vi "CSTK_Icon_Creator_Insert_UpdateImageData.vi"(6 "图片数据输入":T1, 8 "error in (no error)":errorcluster, 11 "图片输入":picture) -> (0 "error out":errorcluster, 3 "图片输出":picture, 4 "图片数据输出":T1)   [LabVIEW 2015, in "CSTK_Icon Creator.lvlib"]
uses:
  CSTK_Icon Creator.lvlib
  <vilib>/picture/picture.llb/imagedata.ctl
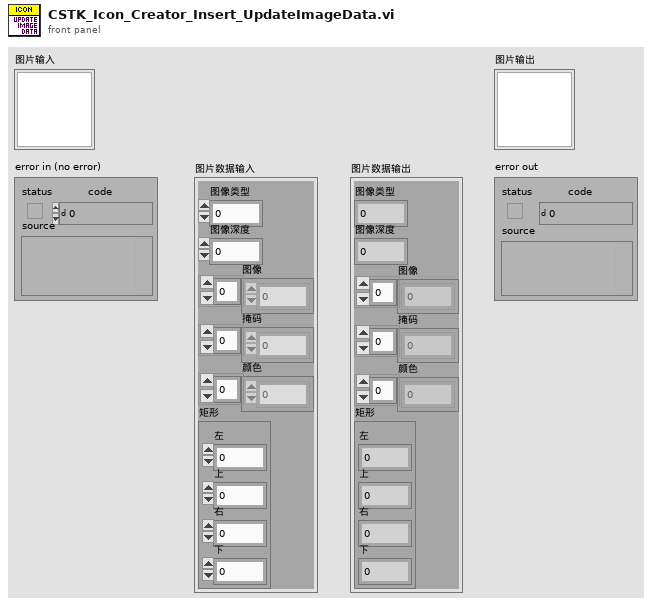
[diagram p1: front panel]
types:
  T1 = typedef "imagedata.ctl" = cluster{"image type":i32, "image depth":i32, "image":u8[], "mask":u8[], "colors":u32[], "Rectangle":cluster{"left":i16, "top":i16, "right":i16, "bottom":i16}}
  T2 = cluster{"left":i16, "top":i16, "right":i16, "bottom":i16}
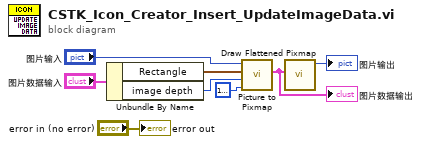
[diagram p0: block diagram]
diagram:
  n1 = Unbundle By Name("图片数据输入") -> ("Rectangle"=w7:T2, "image depth"=w6:i32)
  n2 = call <vilib>:"Picture to Pixmap.vi"("Background Color"=u32 16777216, "depth"=w6, "rect"=w7, "picture"="图片输入") -> ("image data"=w4:T1)  [unwired: 6 in, 1 out]
  "图片数据输出" <- w4
  n3 = call <vilib>:"Draw Flattened Pixmap.vi"("image data"=w4) -> ("new picture"=→"图片输出":picture)  [unwired: 8 in]
  "error out" <- "error in (no error)"
